vi "SaveBodyCameraImage.vi"(5 "Save Format":enum16{"Png", "Raw"}(ring), 7 "Save Image?":bool, 8 "Block Folder":path, 9 "Subfolder":string="Eyetracker", 10 "Refnum in":T1) -> (2 "Refnum out (duplicate)":T1, 3 "ImageSaved":bool=TRUE)   [LabVIEW 2013]
uses:
  <vilib>/vision/Image Controls.llb/IMAQ Image.ctl
  <vilib>/Utility/file.llb/Write To Spreadsheet File (string).vi
  <vilib>/vision/NI_Vision_Development_Module.lvlib
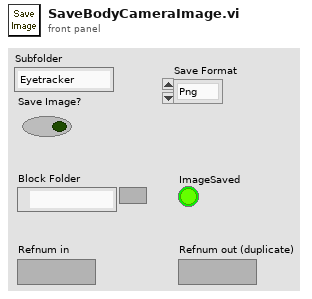
[diagram p1: front panel]
types:
  T1 = typedef "IMAQ Image.ctl" = refnum<image>
  T2 = enum16{"open", "replace", "create", "open or create", "replace or create", "replace or create with confirmation"}
  T3 = cluster{"Desired Font (Application)":enum16{"User-specified Font", "Application Font", "System Font", "Dialog Font"}, "[User-specified Font]":cluster{"Font Name":string, "Size":i16, "Strikeout?":bool, "Italic?":bool, "Underline?":bool, "Outline?":bool, "Shadow?":bool, "Bold?":bool, "Rotation Angle":dbl}, "Horizontal Alignment":i16, "Vertical Alignment":i16}
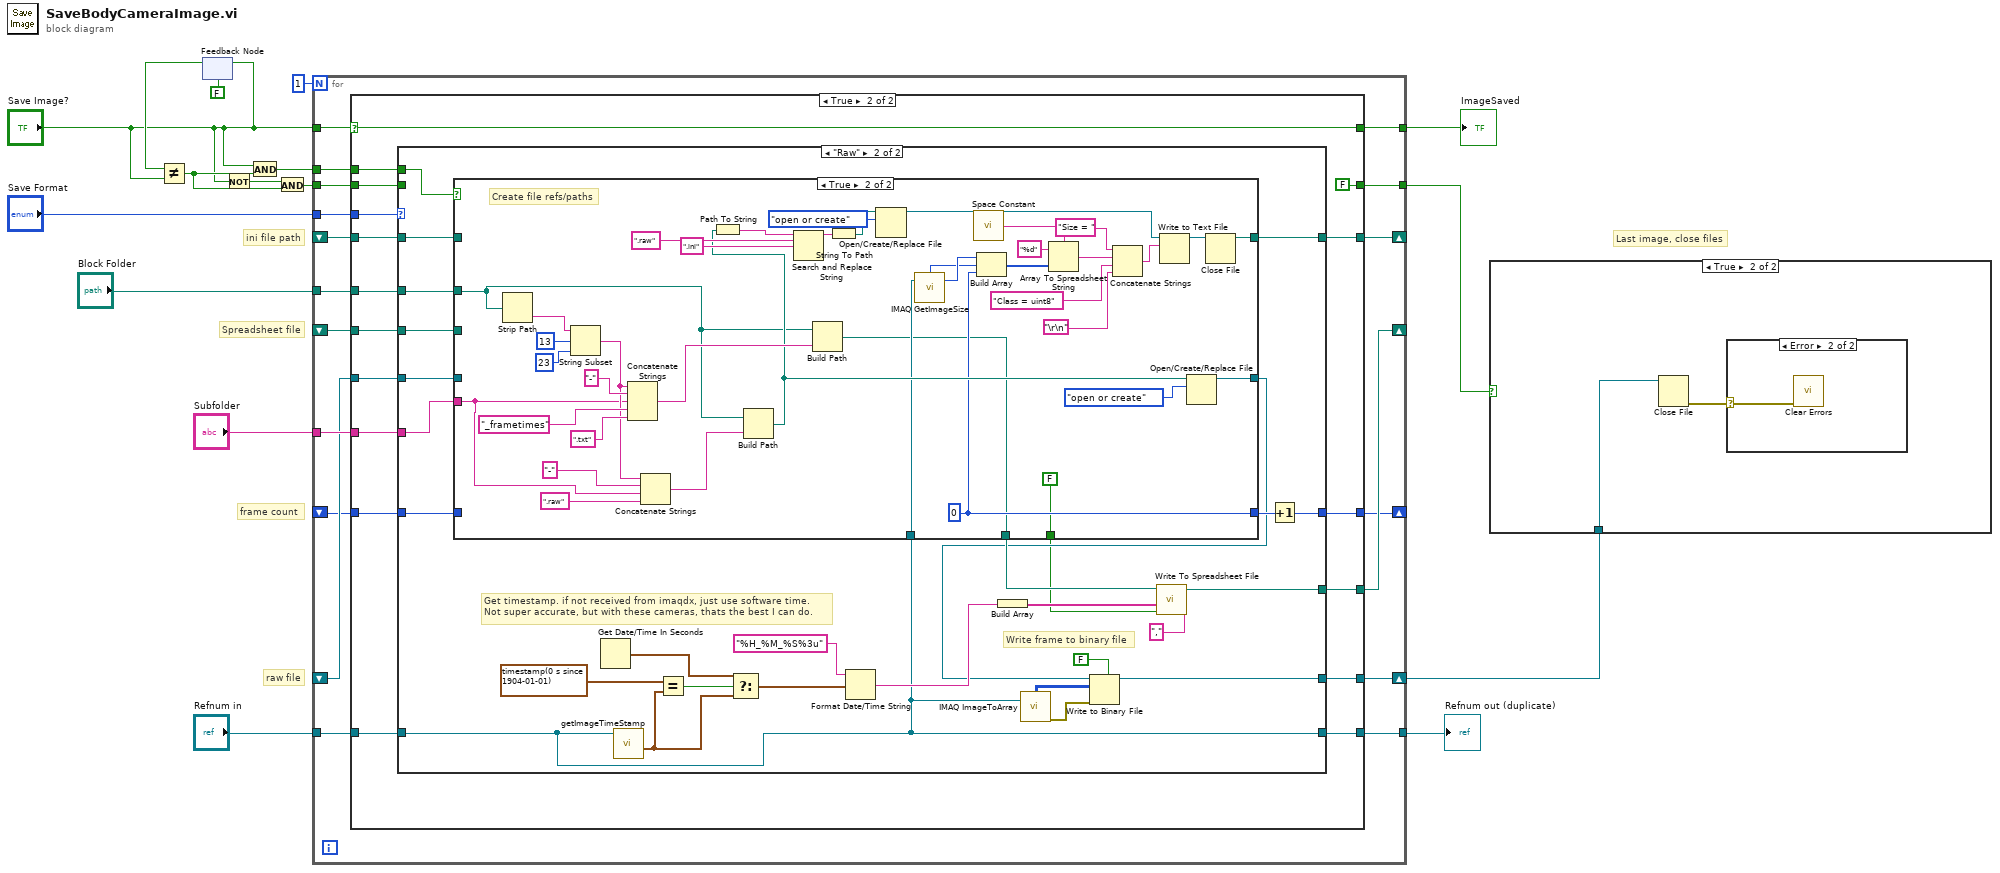
[diagram p0: block diagram]
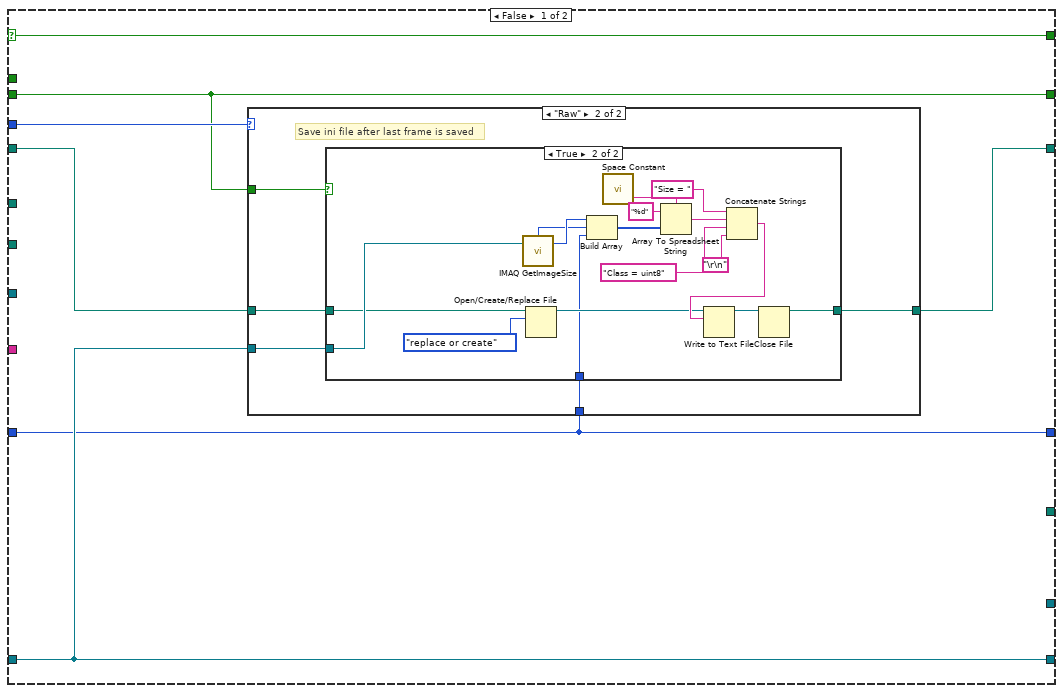
[diagram p4: hidden frame]
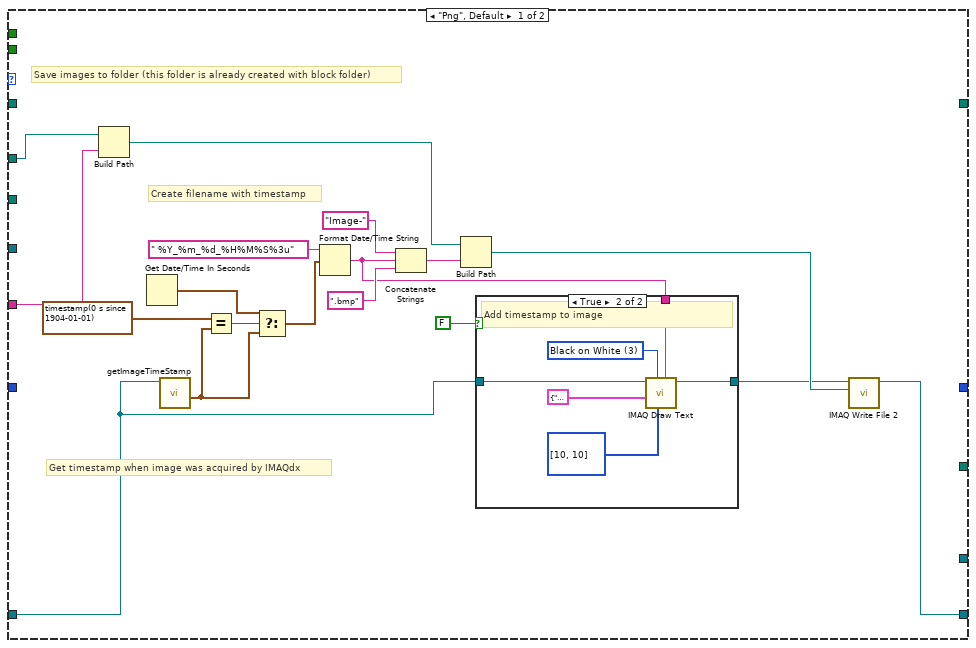
[diagram p7: hidden frame]
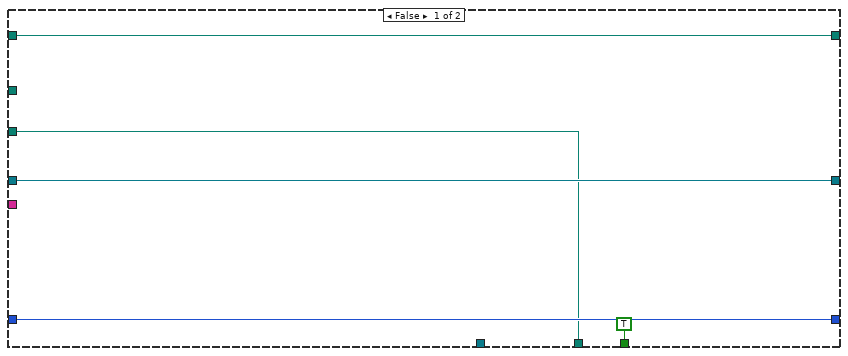
[diagram p9: hidden frame]
diagram:
  # "frame count"
  # "Spreadsheet file"
  # "raw file"
  # "ini file path"
  # "Last image, close files"
  n1 = feedback-in #1("Save Image?") -> ()
  n2 = feedback #1(FALSE ("Save Image?")) -> (w4:bool)
  n3 = Not Equal?(x=w4, y="Save Image?") -> (x != y?=w3:bool)
  n4 = Not(x="Save Image?") -> (.not. x?=w2:bool)
  n5 = And(x="Save Image?", y=w3) -> (x .and. y?=w6:bool)
  n6 = And(x=w2, y=w3) -> (x .and. y?=w5:bool)
  n7 = for {
    N: 1 -> [_]
    tunnel: [w34] -> w16
    tunnel: "Block Folder" -> [w33]
    tunnel: "Refnum in" -> [w32]
    tunnel: "Save Image?" -> [w31]
    tunnel: [w30] -> w10
    tunnel: "Subfolder" -> [w29]
    tunnel: "Save Format" -> [w28]
    tunnel: w6 -> [w27]
    shift-right: [w26] -> _
    shift-left: _ -> [w25]
    shift-right: [w24] -> w8
    shift-left: _ -> [w23]
    tunnel: w5 -> [w22]
    shift-right: [w21] -> _
    shift-left: _ -> [w20]
    tunnel: [w19] -> w9
    shift-right: [w18] -> _
    shift-left: _ -> [w17]
    n8 = case shown="True" w31 {
      selector: w31 -> [w41 w79]
      tunnel: [w39 w81] -> w34
      tunnel: w33 -> [_ w82]
      tunnel: w32 -> [w39 w80]
      tunnel: [w41 w79] -> w30
      tunnel: w29 -> [_ w78]
      tunnel: w28 -> [w40 w77]
      tunnel: w27 -> [_ w76]
      tunnel: [_ w75] -> w24
      tunnel: [_ w74] -> w26
      tunnel: w25 -> [_ w73]
      tunnel: w23 -> [_ w72]
      tunnel: w22 -> [w35 w71]
      tunnel: [w38 w70] -> w21
      tunnel: w20 -> [w38 w69]
      tunnel: [w35 FALSE ("Last Frame")] -> w19
      tunnel: [w36 w67] -> w18
      tunnel: w17 -> [w37 w66]
      frame False {
        n9 = case shown="\"Raw\"" w40 {
          tunnel: w39 -> [_ w47]
          tunnel: w38 -> [_ w46]
          tunnel: w37 -> [w42 w45]
          tunnel: [w42 w44] -> w36
          tunnel: w35 -> [_ w43]
          frame "Png", Default {
          }
          frame "Raw" {
            # "Save ini file after last frame is saved"
            n10 = case shown="True" w43 {
              tunnel: w47 -> [_ w57]
              tunnel: w46 -> [_ w55]
              tunnel: w45 -> [w48 w53]
              tunnel: [w48 w52] -> w44
              frame False {
              }
              frame True {
                n11 = call "IMAQ GetImageSize"("Image"=w57) -> ("Y Resolution"=w65:i32, "X Resolution"=w64:i32)  [unwired: 3 in, 1 out]
                n12 = Open/Create/Replace File(file path (use dialog)=w53, operation (0:open)=T2."replace or create") -> (refnum out=w56:refnum<file>)  [unwired: 4 in, 2 out]
                n13 = Build Array(w65, w64, w55) -> (w63:i32[])
                n14 = call <vilib>:"Space Constant.vi"() -> ("String"=w51:string)
                n15 = Array To Spreadsheet String(delimiter (Tab)=w51, array=w63, 3:"%d" ("format string")) -> (spreadsheet string=w61:string)
                n16 = Concatenate Strings("Size = " ("string"), w61, "Class = uint8" ("string"), "\r\n") -> (w58:string)
                n17 = Write to Text File(file (use dialog)=w56, text=w58) -> (refnum out=w59:refnum<file>)  [unwired: 2 in, 2 out]
                n18 = Close File(refnum=w59) -> (path=w52:path)  [unwired: 1 in, 1 out]
              }
            }
          }
        }
      }
      frame True {
        n19 = case shown="\"Raw\"" w77 {
          tunnel: w82 -> [w95 w121]
          tunnel: [w92 w108] -> w81
          tunnel: w80 -> [w90 w108]
          tunnel: w78 -> [w88 w122]
          tunnel: w76 -> [_ w115]
          tunnel: [_ w123] -> w75
          tunnel: [_ w120] -> w74
          tunnel: w73 -> [_ w119]
          tunnel: w72 -> [_ w118]
          tunnel: w71 -> [_ _]
          tunnel: [_ w116] -> w70
          tunnel: w69 -> [_ w117]
          tunnel: [_ w113] -> w67
          tunnel: w66 -> [_ w111]
          frame "Png", Default {
            # "Get timestamp when image was acquired by IMAQdx"
            # "Save images to folder (this folder is already created with block folder)"
            # "Create filename with timestamp"
            n20 = Build Path(base path=w95, name or relative path=w88) -> (appended path=w94:path)
            n21 = Get Date/Time In Seconds() -> (seconds since 1Jan1904=w86:timestamp)
            n22 = call "getImageTimeStamp.vi"("Image refnum in"=w90) -> ("System Time Stamp"=w85:timestamp)  [unwired: 9 in, 1 out]
            n23 = Equal?(x=timestamp(0 s since 1904-01-01), y=w85) -> (x = y?=w87:bool)
            n24 = Select(t=w86, s=w87, f=w85) -> (s? t:f=w84:timestamp)
            n25 = Format Date/Time String(time format string (%c)=" %Y_%m_%d_%H%M%S%3u", seconds (now)=w84) -> (date/time string=w93:string)  [unwired: 1 in]
            n26 = Concatenate Strings("Image-" ("string"), w93, ".bmp" ("string")) -> (w99:string)
            n27 = Build Path(base path=w94, name or relative path=w99) -> (appended path=w100:path)
            n28 = case shown="True" FALSE {
              tunnel: w93 -> [_ w107]
              tunnel: w90 -> [w101 w103]
              tunnel: [w101 w102] -> w89
              frame False {
              }
              frame True {
                w104 = 3 items=["White", "Black", "Inverted", "Black on White", "White on Black"] ("Color")
                # "Add timestamp to image"
                n29 = call "IMAQ Draw Text"("String"=w107, "Insertion Point"=i32[] [10, 10], "Color"=w104, "Font, Size & Style"=T3 {"Desired Font (Application)"=enum."User-specified Font", "[User-specified Font]"={"Font Name"="", "Size"=26, "Strikeout?"=FALSE, "Italic?"=FALSE, "Underline?"=FALSE, "Outline?"=FALSE, "Shadow?"=FALSE, "Bold?"=FALSE, "Rotation Angle"=0.0}, "Horizontal Alignment"=0, "Vertical Alignment"=1}, "Image Src"=w103) -> ("Image Dst Out"=w102:T1)  [unwired: 3 in, 3 out]
              }
            }
            n30 = call-poly "IMAQ Write File 2"("File Path"=w100, "Image"=w89) -> ("Image Out (duplicate)"=w92:T1)  [unwired: 8 in, 1 out]
          }
          frame "Raw" {
            # "Write frame to binary file"
            # "Get timestamp. if not received from imaqdx, just use software time. \nNot super accurate, but with these cameras, thats the best I can do."
            n31 = case shown="True" w115 {
              tunnel: w122 -> [_ w166]
              tunnel: w121 -> [_ w145]
              tunnel: w119 -> [w138 _]
              tunnel: [w140 w167] -> w110
              tunnel: w118 -> [w140 _]
              tunnel: [w139 w147] -> w114
              tunnel: w117 -> [w139 _]
              tunnel: [w137 w150] -> w113
              tunnel: w108 -> [_ w148]
              tunnel: [w138 w146] -> w112
              tunnel: w111 -> [w137 _]
              tunnel: [TRUE FALSE] -> w109
              frame False {
              }
              frame True {
                w147 = 0
                # "Create file refs/paths"
                n32 = Strip Path(path=w145) -> (name=w175:string)  [unwired: 1 out]
                n33 = String Subset(string=w175, offset (0)=13, length (rest)=23 ("length (rest)")) -> (substring=w170:string)
                n34 = Concatenate Strings(w170, "-" ("string"), w166, "_frametimes" ("string"), ".txt" ("string")) -> (w179:string)
                n35 = Concatenate Strings(w170, "-" ("string"), w166, ".raw" ("string")) -> (w169:string)
                n36 = Build Path(base path=w145, name or relative path=w169) -> (appended path=w161:path)
                n37 = Path To String(path=w161) -> (string=w162:string)
                n38 = Search and Replace String(input string=w162, search string=".raw", replace string=".ini" ("replace string (\"\")")) -> (result string=w165:string)  [unwired: 5 in, 3 out]
                n39 = Build Path(base path=w145, name or relative path=w179) -> (appended path=w146:path)
                n40 = String To Path(string=w165) -> (path=w160:path)
                n41 = Open/Create/Replace File(file path (use dialog)=w160, operation (0:open)=T2."open or create") -> (refnum out=w149:refnum<file>)  [unwired: 4 in, 2 out]
                n42 = call "IMAQ GetImageSize"("Image"=w148) -> ("Y Resolution"=w158:i32, "X Resolution"=w157:i32)  [unwired: 3 in, 1 out]
                n43 = call <vilib>:"Space Constant.vi"() -> ("String"=w143:string)
                n44 = Build Array(w158, w157, w147) -> (w156:i32[])
                n45 = Array To Spreadsheet String(delimiter (Tab)=w143, array=w156, 3:"%d" ("format string")) -> (spreadsheet string=w154:string)
                n46 = Concatenate Strings("Size = " ("string"), w154, "Class = uint8" ("string"), "\r\n") -> (w151:string)
                n47 = Write to Text File(file (use dialog)=w149, text=w151) -> (refnum out=w152:refnum<file>)  [unwired: 2 in, 2 out]
                n48 = Open/Create/Replace File(file path (use dialog)=w161, operation (0:open)=T2."open or create") -> (refnum out=w167:refnum<file>)  [unwired: 4 in, 2 out]
                n49 = Close File(refnum=w152) -> (path=w150:path)  [unwired: 1 in, 1 out]
              }
            }
            n50 = Get Date/Time In Seconds() -> (seconds since 1Jan1904=w133:timestamp)
            n51 = call "getImageTimeStamp.vi"("Image refnum in"=w108) -> ("System Time Stamp"=w130:timestamp)  [unwired: 9 in, 1 out]
            n52 = Equal?(x=timestamp(0 s since 1904-01-01), y=w130) -> (x = y?=w134:bool)
            n53 = Select(t=w133, s=w134, f=w130) -> (s? t:f=w132:timestamp)
            n54 = Format Date/Time String(time format string (%c)="%H_%M_%S%3u", seconds (now)=w132) -> (date/time string=w125:string)  [unwired: 1 in]
            n55 = Build Array(w125) -> (w124:string[])
            n56 = call "IMAQ ImageToArray"("Image"=w108) -> ("error out"=w128:errorcluster, "Image Pixels (U8)"=w127:u8[][])  [unwired: 3 in, 3 out]
            n57 = Write to Binary File(file (use dialog)=w110, data=w127, error in=w128, 5:FALSE ("prepend array or string size? (T)")) -> (refnum out=w123:refnum<file>)  [unwired: 2 in, 2 out]
            n58 = call-poly <vilib>:"Write To Spreadsheet File.vi"("delimiter (\\t)"="," ("delimiter (\\t)"), "append to file? (new file:F)"=w109, "1D data"=w124, "file path (dialog if empty)"=w112) -> ("new file path (Not A Path if cancelled)"=w120:path)  [unwired: 3 in, 1 out]
            n59 = Increment(x=w114) -> (x+1=w116:i32)
          }
        }
      }
    }
  }
  "Refnum out (duplicate)" <- w16
  "ImageSaved" <- w10
  n60 = case shown="True" w9 {
    tunnel: w8 -> [_ w181]
    frame False {
    }
    frame True {
      n61 = Close File(refnum=w181) -> (error out=w180:errorcluster)  [unwired: 1 in, 1 out]
      n62 = case shown="Error" w180 {
        selector: w180 -> [_ w182]
        frame No Error {
        }
        frame Error {
          n63 = call <vilib>:"Clear Errors.vi"("error in (no error)"=w182) -> ()  [unwired: 6 in, 1 out]
        }
      }
    }
  }
